vi "Columns.vi"() -> (2 "Columns":T1)   [LabVIEW 2020, in "NewEntityTemplate.lvclass"]
uses:
  NewEntityTemplate.lvclass
  Columns.ctl
  Conditum/Columns/Integer/Integer.lvclass
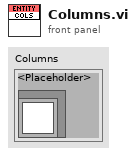
[diagram p1: front panel]
types:
  T1 = typedef "NewEntityTemplate.lvclass/Columns.ctl" = cluster{"<Placeholder>":refnum<class "Integer.lvclass">}
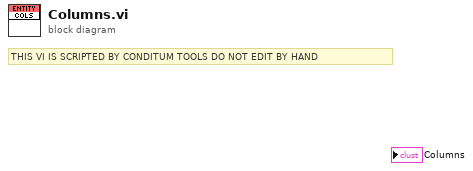
[diagram p0: block diagram]
diagram:
  # "THIS VI IS SCRIPTED BY CONDITUM TOOLS DO NOT EDIT BY HAND"
